vi "Info.vi"(4 "Message":string, 6 "Source":string, 8 "error in (no error)":errorcluster) -> (0 "error out":errorcluster)   [LabVIEW 2024, in "RQMHLogger.lvlib"]
uses:
  RQMHLogger.lvlib
  RQMHLogger/RQMHLogger.lvclass
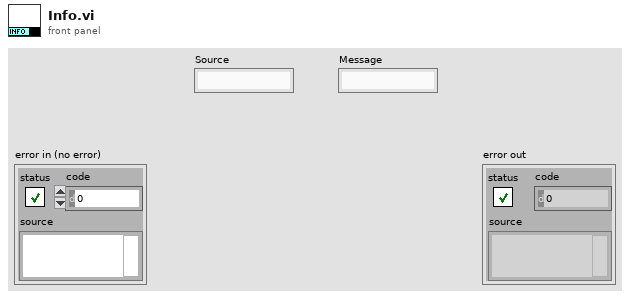
[diagram p1: front panel]
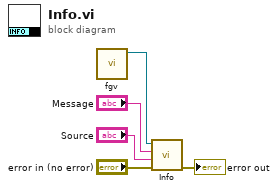
[diagram p0: block diagram]
diagram:
  n1 = call "fgv.vi"() -> ("RQMHLogger Get"=w5:refnum<class "RQMHLogger.lvclass">)  [unwired: 11 in]
  n2 = call "Info.vi"("error in (no error)"="error in (no error)", "Source"="Source", "Message"="Message", "RQMHLogger in"=w5) -> ("error out"=→"error out":errorcluster)  [unwired: 6 in, 1 out]
